vi "Animate To Size & Position.vi"(5 "Delay mS":u32, 7 "Steps":i32, 8 "Callback Owner":refnum<class>, 9 "Done Callback":refnum<vi>, 10 "Dest Bounds":T1, 11 "VI Refnum":refnum<vi>) -> ()   [LabVIEW 2020, in "PicoG-Processor.lvlib"]
uses:
  PicoG-Processor.lvlib
  <vilib>/Utility/miscctls.llb/LVRectTypeDef.ctl
  _Animate to Size & Position.vi
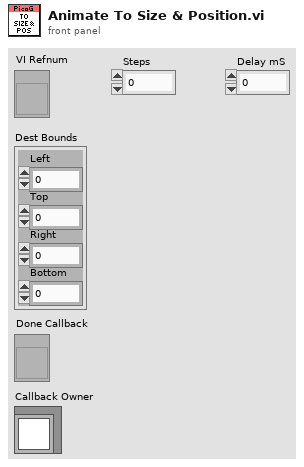
[diagram p1: front panel]
types:
  T1 = typedef "LVRectTypeDef.ctl" = cluster{"Left":i16, "Top":i16, "Right":i16, "Bottom":i16}
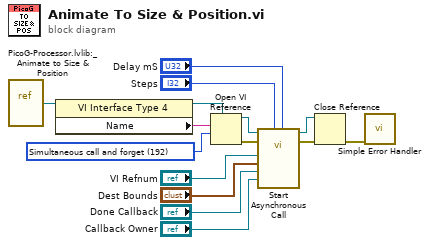
[diagram p0: block diagram]
diagram:
  w10 = 192 items=["Record modifications"=1, "Open templates for editing"=2, "Prompt user to save"=4, "Prepare for reentrant run"=8, "Prompt to find missing subVIs"=16, "Hide loading dialog box"=32, "Enable simultaneous calls"=64, "Prepare to call and forget"=128, "Simultaneous call and forget"=192, "Prepare to call and collect"=256, "Simultaneous call and collect"=320]
  n1 = vi-ref "PicoG-Processor.lvlib:_Animate to Size & Position.vi"() -> (w8:refnum<vi>)
  n2 = property class="VI Interface Type 4"(reference=w8) -> (reference out=w11:refnum<vi>, "Name"=w9:string)  [unwired: 1 in, 1 out]
  n3 = Open VI Reference(type specifier VI Refnum (for type only)=w11, vi path=w9, options=w10) -> (vi reference=w13:refnum<vi>, error out=w12:errorcluster)  [unwired: 3 in]
  n4 = call-by-ref "Start Asynchronous Call"(reference=w13, error in=w12, "Delay mS"="Delay mS", "Steps"="Steps", "Callback Owner"="Callback Owner", "Done Callback"="Done Callback", "Dest Bounds"="Dest Bounds", "VI Refnum"="VI Refnum") -> (reference out=w15:refnum<vi>, error out=w14:errorcluster)  [unwired: 6 in]
  n5 = Close Reference(reference=w15, error in (no error)=w14) -> (error out=w3:errorcluster)
  n6 = call <vilib>:"Simple Error Handler.vi"("error in (no error)"=w3) -> ()  [unwired: 4 in, 5 out]
